vi "Localization.vi"(7 "section":T1, 8 "error in (no error)":errorcluster, 10 "key":string[](array[string]), 11 "Language key":string) -> (0 "error out":errorcluster, 3 "Value":string[](array[string]))   [LabVIEW 2025, in "Localization.lvlib"]
uses:
  Localization.lvlib
  Section.ctl
  <vilib>/Utility/config.llb/Read Key (String).vi
  <vilib>/Utility/config.llb/NI_LVConfig.lvlib
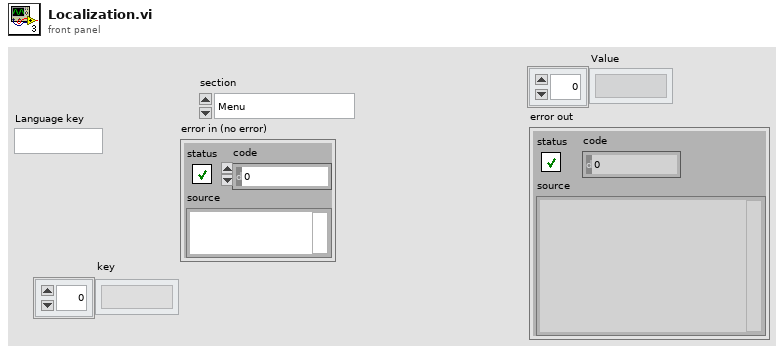
[diagram p1: front panel]
types:
  T1 = typedef "Localization.lvlib/Section.ctl" = enum16{"Menu", "Title", "Workstation Config"}
  T2 = typedef "NI_LVConfig.lvlib/Config Data RefNum.ctl" = refnum<k1>
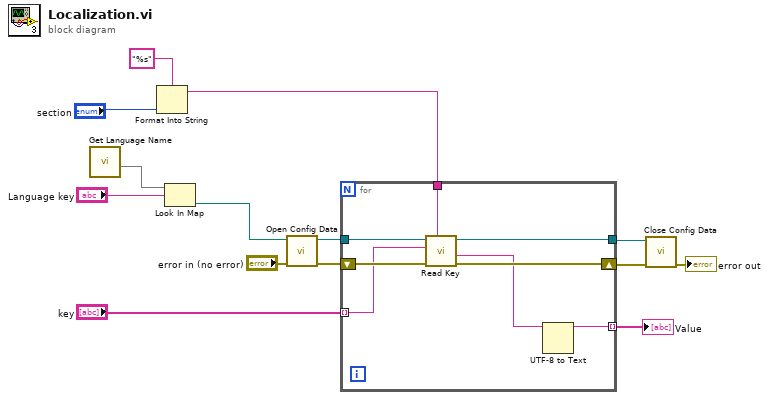
[diagram p0: block diagram]
diagram:
  n1 = call "Get Language Name.vi"() -> ("Path"=w14:map{string, path})  [unwired: 8 in, 3 out]
  n2 = Format Into String(format string="%s", "section") -> (resulting string=w7:string)  [unwired: 2 in, 1 out]
  n3 = Look In Map(map=w14, key="Language key") -> (value=w12:path)  [unwired: 1 in, 1 out]
  n4 = call <vilib>:"Open Config Data.vi"("error in (no error)"="error in (no error)", "configuration file path"=w12) -> ("error out"=w10:errorcluster, "refnum"=w11:T2)  [unwired: 7 in, 1 out]
  n5 = for {
    tunnel: w11 -> [w22]
    tunnel: w7 -> [w20]
    tunnel: [w19] -> w3
    shift-right: [w18] -> w2
    shift-left: w10 -> [w21]
    tunnel: "key" -> [w17] mode=indexing
    tunnel: [w15] -> w4 mode=indexing
    n6 = call-poly <vilib>:"Read Key.vi"("section"=w20, "error in (no error)"=w21, "key"=w17, "refnum"=w22) -> ("error out"=w18:errorcluster, "value"=w16:string, "refnum out"=w19:T2)  [unwired: 4 in, 1 out]
    n7 = UTF-8 to Text(11:w16) -> (3:w15:string)  [unwired: 2 in, 1 out]
  }
  "Value" <- w4
  n8 = call <vilib>:"Close Config Data.vi"("error in (no error)"=w2, "refnum"=w3) -> ("error out"=→"error out":errorcluster)  [unwired: 8 in, 1 out]
